vi "Assignment1_Speedometer.vi"() -> ()   [LabVIEW 2024]
panel:
  out "km/h":dbl(knob) scale=0.0..160.0
  in  "miles/h":dbl(knob) scale=0.0..100.0
  out "String":string
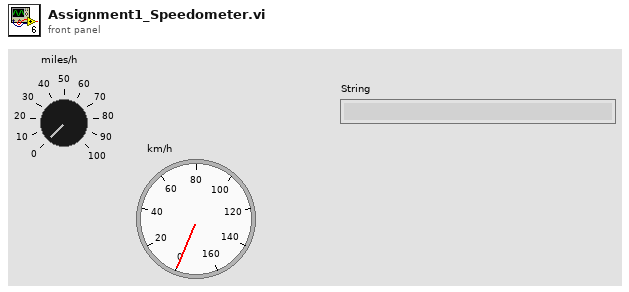
[diagram p1: front panel]
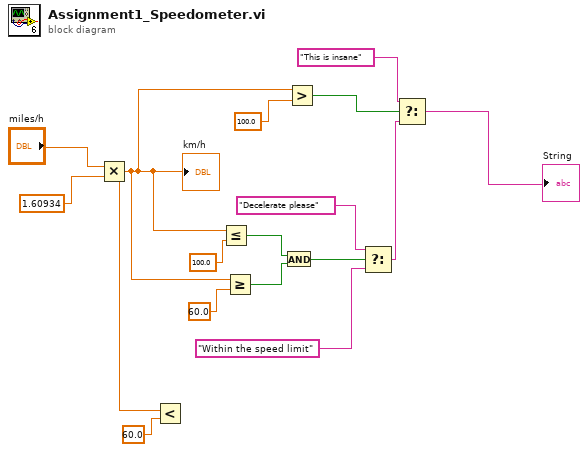
[diagram p0: block diagram]
diagram:
  n1 = Multiply(x="miles/h", y=1.60934) -> (x*y=w1:dbl)
  "km/h" <- w1
  n2 = Less?(x=w1, y=60.0) -> ()  [unwired: 1 out]
  n3 = Less Or Equal?(x=w1, y=100.0) -> (x <= y?=w12:bool)
  n4 = Greater Or Equal?(x=w1, y=60.0) -> (x >= y?=w11:bool)
  n5 = And(x=w12, y=w11) -> (x .and. y?=w5:bool)
  n6 = Greater?(x=w1, y=100.0) -> (0:w9:bool)
  n7 = Select(t="Decelerate please", s=w5, f="Within the speed limit") -> (s? t:f=w4:string)
  n8 = Select(t="This is insane", s=w9, f=w4) -> (s? t:f=→"String":string)
